vi "Remote PC - Client.vi"(6 "Remote Sever Port (2800)":u16, 7 "Flow Contorl":enum16{"Connect", "Read", "Write", "Close"}(ring), 8 "error in":errorcluster, 9 "Send Command":T1, 11 "IP Address":string) -> (0 "error out":errorcluster, 1 "Receive Message":string)   [LabVIEW 2012]
uses:
  TypeDef/Send Command Message.ctl
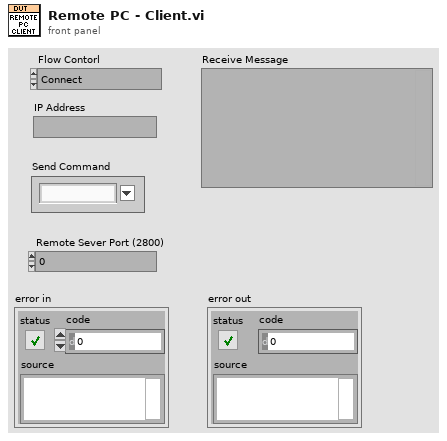
[diagram p1: front panel]
types:
  T1 = typedef "Send Command Message.ctl" = string
  T2 = enum16{"Standard", "Buffered", "CRLF", "Immediate"}
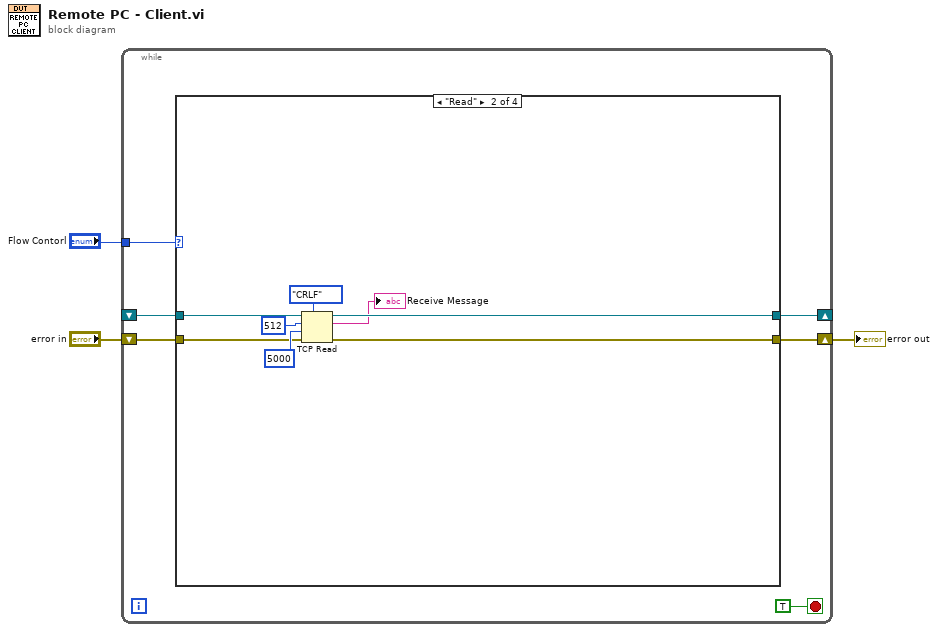
[diagram p0: block diagram]
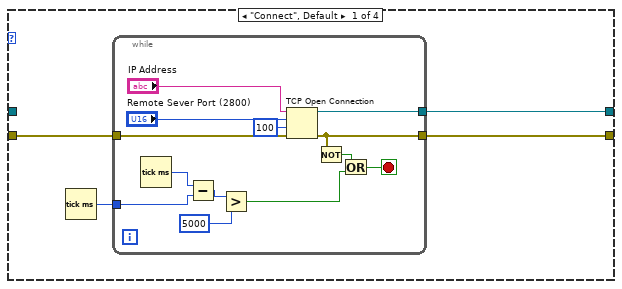
[diagram p2: hidden frame]
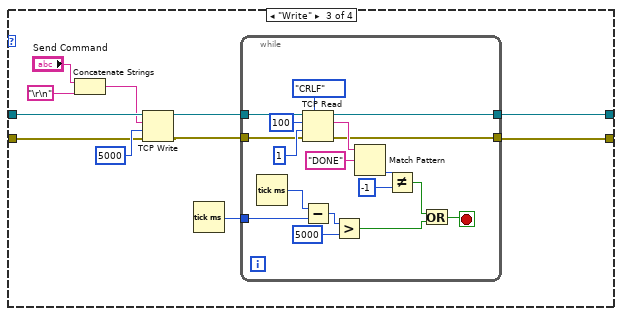
[diagram p3: hidden frame]
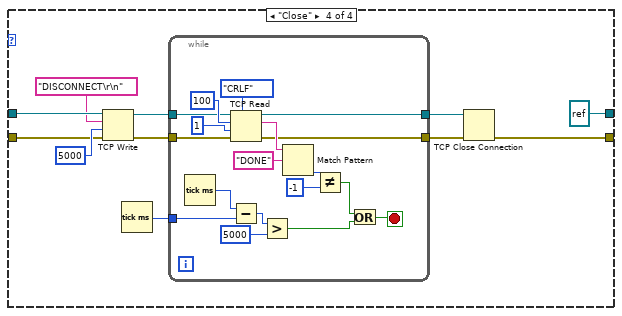
[diagram p4: hidden frame]
diagram:
  n1 = while {
    shift-right: [w7] -> w2
    shift-left: "error in" -> [w8]
    shift-right: [w6] -> _
    shift-left: _ -> [w5]
    tunnel: "Flow Contorl" -> [w4]
    stop <- TRUE stop-if-true
    n2 = case shown="\"Read\"" w4 {
      tunnel: w8 -> [w13 w30 w43 w71]
      tunnel: [w12 w29 w38 w74] -> w7
      tunnel: [w11 w28 w39 refnum<k5> refnum ("connection ID")] -> w6
      tunnel: w5 -> [_ w31 w44 w70]
      frame "Connect", Default {
        n3 = Tick Count (ms)() -> (millisecond timer value=w10:u32)
        n4 = while {
          tunnel: w13 -> [w24]
          tunnel: [w15] -> w12
          tunnel: [w23] -> w11
          tunnel: w10 -> [w20]
          stop <- w16 stop-if-true
          n5 = Tick Count (ms)() -> (millisecond timer value=w21:u32)
          n6 = Subtract(x=w21, y=w20) -> (x-y=w19:u32)
          n7 = Greater?(x=w19, y=u32 5000) -> (0:w17:bool)
          n8 = TCP Open Connection(address="IP Address", remote port or service name="Remote Sever Port (2800)", timeout ms (60000)=100, error in (no error)=w24) -> (connection ID=w23:refnum<k5>, error out=w15:errorcluster)  [unwired: 1 in]
          n9 = Not(x=w15) -> (.not. x?=w14:bool)
          n10 = Or(x=w14, y=w17) -> (x .or. y?=w16:bool)
        }
      }
      frame "Read" {
        n11 = TCP Read(connection ID=w31, bytes to read=512, error in (no error)=w30, 7:T2."CRLF" ("mode (standard)"), 9:5000 ("timeout ms (25000)")) -> (connection ID out=w28:refnum<k5>, data out=→"Receive Message":string, error out=w29:errorcluster)
      }
      frame "Write" {
        n12 = Concatenate Strings("Send Command", "\r\n") -> (w35:string)
        n13 = TCP Write(connection ID=w44, data in=w35, error in (no error)=w43, 9:5000 ("timeout ms (25000)")) -> (connection ID out=w40:refnum<k5>, error out=w41:errorcluster)  [unwired: 1 out]
        n14 = Tick Count (ms)() -> (millisecond timer value=w42:u32)
        n15 = while {
          tunnel: w42 -> [w55]
          tunnel: [w49] -> w39
          tunnel: [w48] -> w38
          tunnel: w40 -> [w47]
          tunnel: w41 -> [w46]
          stop <- w50 stop-if-true
          n16 = Tick Count (ms)() -> (millisecond timer value=w56:u32)
          n17 = TCP Read(connection ID=w47, bytes to read=100, error in (no error)=w46, 7:T2."CRLF" ("mode (standard)"), 9:1 ("timeout ms (25000)")) -> (connection ID out=w49:refnum<k5>, data out=w61:string, error out=w48:errorcluster)
          n18 = Subtract(x=w56, y=w55) -> (x-y=w54:u32)
          n19 = Greater?(x=w54, y=u32 5000) -> (0:w51:bool)
          n20 = Match Pattern(string=w61, regular expression="DONE") -> (offset past match=w59:i32)  [unwired: 1 in, 3 out]
          n21 = Not Equal?(x=w59, y=-1) -> (x != y?=w52:bool)
          n22 = Or(x=w52, y=w51) -> (x .or. y?=w50:bool)
        }
      }
      frame "Close" {
        n23 = TCP Write(connection ID=w70, data in="DISCONNECT\r\n", error in (no error)=w71, 9:5000 ("timeout ms (25000)")) -> (connection ID out=w65:refnum<k5>, error out=w64:errorcluster)  [unwired: 1 out]
        n24 = Tick Count (ms)() -> (millisecond timer value=w68:u32)
        n25 = while {
          tunnel: w68 -> [w84]
          tunnel: [w78] -> w67
          tunnel: [w77] -> w66
          tunnel: w65 -> [w76]
          tunnel: w64 -> [w75]
          stop <- w79 stop-if-true
          n26 = Tick Count (ms)() -> (millisecond timer value=w85:u32)
          n27 = TCP Read(connection ID=w76, bytes to read=100, error in (no error)=w75, 7:T2."CRLF" ("mode (standard)"), 9:1 ("timeout ms (25000)")) -> (connection ID out=w78:refnum<k5>, data out=w90:string, error out=w77:errorcluster)
          n28 = Subtract(x=w85, y=w84) -> (x-y=w83:u32)
          n29 = Greater?(x=w83, y=u32 5000) -> (0:w80:bool)
          n30 = Match Pattern(string=w90, regular expression="DONE") -> (offset past match=w88:i32)  [unwired: 1 in, 3 out]
          n31 = Not Equal?(x=w88, y=-1) -> (x != y?=w81:bool)
          n32 = Or(x=w81, y=w80) -> (x .or. y?=w79:bool)
        }
        n33 = TCP Close Connection(connection ID=w67, error in (no error)=w66) -> (error out=w74:errorcluster)  [unwired: 1 in, 1 out]
      }
    }
  }
  "error out" <- w2
